vi "OutputIntake.vi"   [LabVIEW 2019]
doc: "This VI runs feedback and feedforward control loops, manages safety interlocks, and sends commands to actuators specific to the intake and magazine subsystem."
uses:
  <vilib>/Rock Robotics/WPI/ThirdParty/Phoenix-LabVIEW/Motor Controller/Controls/CTRE_Phoenix_MotorControl_ControlMode.ctl
  <vilib>/Rock Robotics/WPI/Solenoid/WPI_SolenoidValue.ctl
  8b5aedbe-a8a8-4c7c-a5b8-8e231b2757ca.vi
  5ffa2434-d599-47af-b769-9447f6dbdda3.vi
  refnums.vi
  GRNF_CTREMotor.vi
  GRNF_GenericSolenoid.vi
  outputs.vi
  TAI_Motor.vi
  dsdata.vi
  TAI_Solenoid.vi
  <vilib>/Rock Robotics/WPI/Solenoid/WPI_SolenoidSetEnum.vi
types:
  T1 = typedef "CTRE_Phoenix_MotorControl_ControlMode.ctl" = u16
  T2 = typedef "WPI_MotorControlDeviceRef.ctl" = cluster{"DeviceStatus":errorcluster, "Type":T3, "PWM":cluster{"PWM Channel":T4, "DeadBand":T5}, "CAN":cluster{"Device Number":u8, "SetOutput VI Ref":variant, "GetOutput VI Ref":variant, "Enable VI Ref":variant, "Disable VI Ref":variant, "Data":variant}, "Invert":bool, "DIO PWM":cluster{"PWM \"Enable\" Channel":T4, "DIOChannel":T6, "PWM Rate":dbl}}
  T3 = typedef "WPI_MotorControlType.ctl" = enum16{"PWM", "CAN", "DIO PWM"}
  T4 = typedef "FPGA_DIOPWMChannel.ctl" = enum8{"PWM 0", "PWM 1", "PWM 2", "PWM 3", "PWM 4", "PWM 5", "PWM 6", "PWM 7", "PWM 8", "PWM 9", "PWM MXP 0", "PWM MXP 1", "PWM MXP 2", "PWM MXP 3", "PWM MXP 4", "PWM MXP 5", "PWM MXP 6", "PWM MXP 7", "PWM MXP 8", "PWM MXP 9", "Invalid"}
  T5 = typedef "WPI_PWMDeadband.ctl" = cluster{"Name":string, "maxPositivePwm":i32, "minPositivePwm":i32, "centerPwm":i32, "maxNegativePwm":i32, "minNegativePwm":i32, "angularRange":u16}
  T6 = typedef "FPGA_DIOChannel.ctl" = enum8{"DIO 0", "DIO 1", "DIO 2", "DIO 3", "DIO 4", "DIO 5", "DIO 6", "DIO 7", "DIO 8", "DIO 9", "DIO MXP 0", "DIO MXP 1", "DIO MXP 2", "DIO MXP 3", "DIO MXP 4", "DIO MXP 5", "DIO MXP 6", "DIO MXP 7", "DIO MXP 8", "DIO MXP 9", "DIO MXP 10", "DIO MXP 11", "DIO MXP 12", "DIO MXP 13", "DIO MXP 14", "DIO MXP 15", "SPI Port CS1", "SPI Port CS2", "SPI Port CS3", "SPI Port MISO", "SPI Port MOSI", "Invalid"}
  T7 = typedef "WPI_SolenoidDevRef.ctl" = cluster{"DevStatus":errorcluster, "Pneumatics Control Module":u8, "Forward Solenoid Channel":T8, "Reverse Solenoid Channel":T8}
  T8 = typedef "WPI_SolenoidChannel.ctl" = enum8{"Solenoid 0", "Solenoid 1", "Solenoid 2", "Solenoid 3", "Solenoid 4", "Solenoid 5", "Solenoid 6", "Solenoid 7", "Invalid"}
  T9 = typedef "WPI_SolenoidValue.ctl" = enum16{"Off", "On", "Forward", "Reverse"}
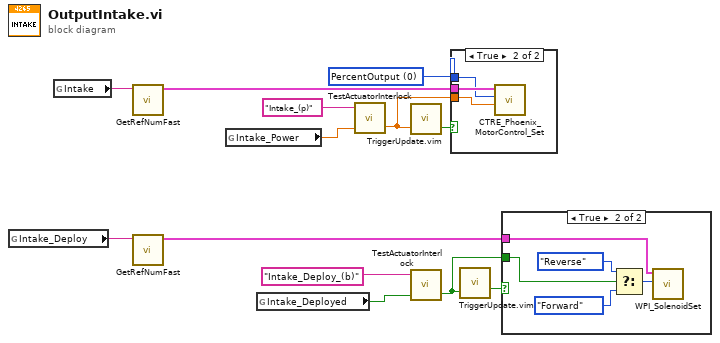
[diagram p0: block diagram]
diagram:
  w1 = T1 0 items=["PercentOutput"=0, "Position"=1, "Velocity"=2, "Current"=3, "Follower"=5, "MotionProfile"=6, "MotionMagic"=7, "MotionProfileArc"=10, "Disabled"=15] ("Control Mode")
  n1 = global read "refnums.vi" "Intake_Deploy"() -> (w8:string)
  n2 = global read "refnums.vi" "Intake"() -> (w9:string)
  n3 = call-poly "GetRefNumFast.vi"("RefNum Name"=w9) -> ("Device Reference"=w11:T2)  [unwired: 5 in, 1 out]
  n4 = call-poly "GetRefNumFast.vi"("RefNum Name"=w8) -> ("Device Reference"=w10:T7)  [unwired: 5 in, 1 out]
  n5 = global read "outputs.vi" "Intake_Power"() -> (w5:dbl)
  n6 = global read "outputs.vi" "Intake_Deployed"() -> (w2:bool)
  n7 = call-poly "TestActuatorInterlock.vi"("Normal Output"=w5, "Actuator Name"="Intake_(p)" ("Actuator_Name")) -> ("Interlock Output"=w7:dbl)  [unwired: 1 in, 1 out]
  n8 = call "TriggerUpdate.vim"("Trigger"=w7) -> ("Update"=w12:bool)  [unwired: 2 in]
  n9 = call-poly "TestActuatorInterlock.vi"("Normal Output"=w2, "Actuator Name"="Intake_Deploy_(b)" ("Actuator_Name")) -> ("Interlock Output"=w3:bool)  [unwired: 1 in, 1 out]
  n10 = case shown="True" w12 {
    tunnel: w11 -> [_ w16]
    tunnel: w7 -> [_ w15]
    tunnel: w1 -> [_ w14]
    frame False {
    }
    frame True {
      n11 = call <vilib>:"CTRE_Phoenix_MotorControl_Set.vi"("Output"=w15, "Control Mode"=w14, "PhoenixMotorControlDevRef"=w16) -> ()  [unwired: 7 in, 2 out]
    }
  }
  n12 = call "TriggerUpdate.vim"("Trigger"=w3) -> ("Update"=w13:bool)  [unwired: 2 in]
  n13 = case shown="True" w13 {
    tunnel: w3 -> [_ w17]
    tunnel: w10 -> [_ w18]
    frame False {
    }
    frame True {
      n14 = Select(t=WPI_SolenoidValue."Reverse" ("Value"), s=w17, f=WPI_SolenoidValue."Forward" ("Value")) -> (s? t:f=w21:T9)
      n15 = call-poly <vilib>:"WPI_SolenoidSet.vi"("Value"=w21, "SolenoidDevRef"=w18) -> ()  [unwired: 8 in, 2 out]
    }
  }
